vi "Add Object Parameter - Numeric.vi"(8 "error in (no error)":errorcluster, 9 "Name":string, 10 "Numeric":dbl, 11 "JSON Tree in (JSON Object)":variant) -> (0 "error out":errorcluster, 3 "JSON Tree out (JSON Object)":variant)   [LabVIEW 2011, in "i3-json.lvlib"]
doc: "Use this template to build a VI to use as a subVI."
uses:
  i3-json.lvlib
  JSON Types/JSON Type.ctl
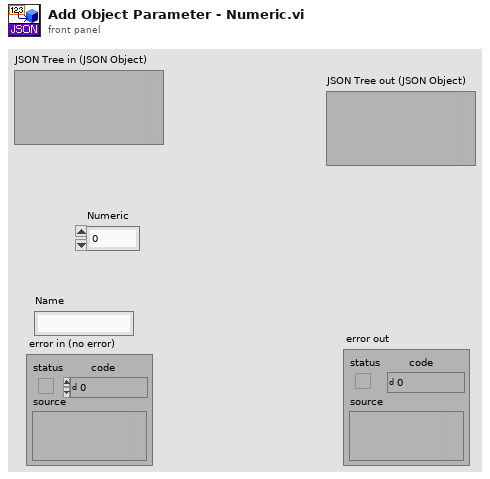
[diagram p1: front panel]
types:
  T1 = typedef "i3-json.lvlib/JSON Type.ctl" = enum8{"JSON Compatible", "JSON Array", "JSON Object", "JSON Null", "Double", "String", "Boolean", "Unknown", "Data JSON string"}
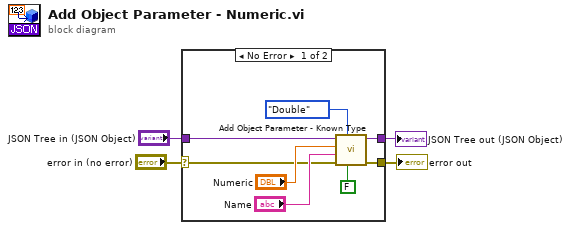
[diagram p0: block diagram]
diagram:
  n1 = case shown="No Error" "error in (no error)" {
    selector: "error in (no error)" -> [w5 w14]
    tunnel: [w12 w14] -> w3
    tunnel: [w11 w13] -> w2
    tunnel: "JSON Tree in (JSON Object)" -> [w10 w13]
    frame No Error {
      n2 = call "Add Object Parameter - Known Type.vi"("Add Parameter as JSON Tree?"=FALSE, "JSON Type"=JSON_Type."Double", "error in (no error)"=w5, "Name"="Name", "Value"="Numeric", "JSON Tree in (JSON Object)"=w10) -> ("error out"=w12:errorcluster, "JSON Tree out (JSON Object)"=w11:variant)  [unwired: 4 in]
    }
    frame Error {
    }
  }
  "error out" <- w3
  "JSON Tree out (JSON Object)" <- w2
